vi "load_single_image.vi"(11 "Path":path) -> (3 "image data":T1)   [LabVIEW 2017]
uses:
  <vilib>/picture/picture.llb/imagedata.ctl
  data_loder/data_loader_single_image/data_loder_single_image.lvclass
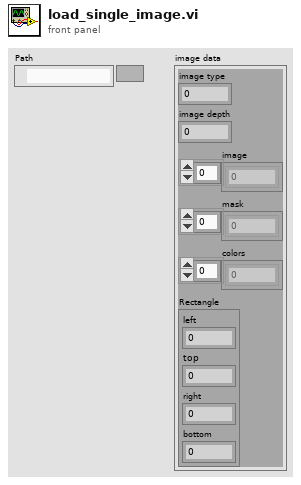
[diagram p1: front panel]
types:
  T1 = typedef "imagedata.ctl" = cluster{"image type":i32, "image depth":i32, "image":u8[], "mask":u8[], "colors":u32[], "Rectangle":cluster{"left":i16, "top":i16, "right":i16, "bottom":i16}}
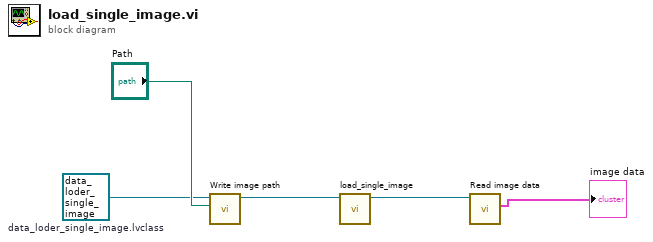
[diagram p0: block diagram]
diagram:
  w1 = refnum<class "data_loder_single_image.lvclass"> refnum  # data_loder_single_image.lvclass
  n1 = call-dynamic "Write image path.vi"("image path"="Path", "data_loder_single_image in"=w1) -> ("data_loder_single_image out"=w3:refnum<class "data_loder_single_image.lvclass">)  [unwired: 8 in, 1 out]
  n2 = call-dynamic "load_single_image.vi"("data_loder_single_image in"=w3) -> ("data_loder_single_image out"=w4:refnum<class "data_loder_single_image.lvclass">)  [unwired: 9 in, 1 out]
  n3 = call-dynamic "Read image data.vi"("data_loder_single_image in"=w4) -> ("image data"=→"image data":T1)  [unwired: 8 in, 2 out]
